vi "CreatePrivateEvents.vi"(8 "error in (no error)":errorcluster, 11 "ParseVectorFile":refnum<class "ParseVectorFile.lvclass">) -> (0 "error out":errorcluster, 3 "ParseVectorFile out":refnum<class "ParseVectorFile.lvclass">)   [LabVIEW 2019, in "ParseVectorFile.lvclass"]
doc: "---------------------------------------------------------------\nJKI State Machine Objects™\nhttp://jki.net/state-machine-objects/\nCopyright (C) 2005-2015, JKI <info@jki.net>\nALL RIGHTS RESERVEDJKI State Machine Objects (SMO) 1.0.0.4\nJKI - JKI\nCopyright (c) 2015, JKI"
uses:
  ParseVectorFile.lvclass
  Typedefs/PrivateEvents--ParseVectorFile.NewFile.ctl
  Typedefs/PrivateEvents--ParseVectorFile.New File Synchronous.ctl
  Typedefs/PublicEvents--ParseVectorFile.ParsedData.ctl
  ParsePaths/Path.lvclass
  Rectangle/Rectangle.lvclass
  Image/SVGImage.lvclass
  Dot/Dot.lvclass
  ParseVectorFile.lvclass/ParseVectorFile.ctl
  <vilib>/JKI/JKI SMO/SMO/SMO.lvclass
panel:
  # "For instructions on how to use the JKI State Machine Objects, examples and video tutorials, visit:\nhttp://jki.net/state-machine-objects/\n\nJKI State Machine Objects™\nhttp://jki.net/state-machine-objects/\nCopyright (C) 2005-2015, JKI <info@jki.net>\nALL RIGHTS RESERVED"
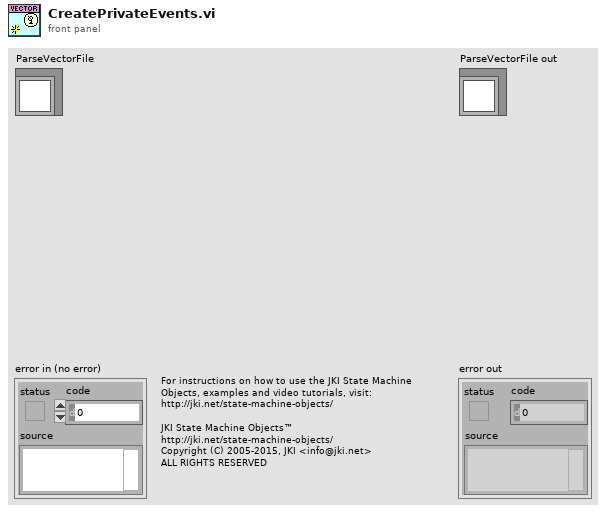
[diagram p1: front panel]
types:
  T1 = typedef "ParseVectorFile.lvclass/PrivateEvents--ParseVectorFile.New File Synchronous.ctl" = cluster{"Path":path, "Parsed Data":refnum<notifier>}
  T2 = typedef "ParseVectorFile.lvclass/PrivateEvents--ParseVectorFile.NewFile.ctl" = path
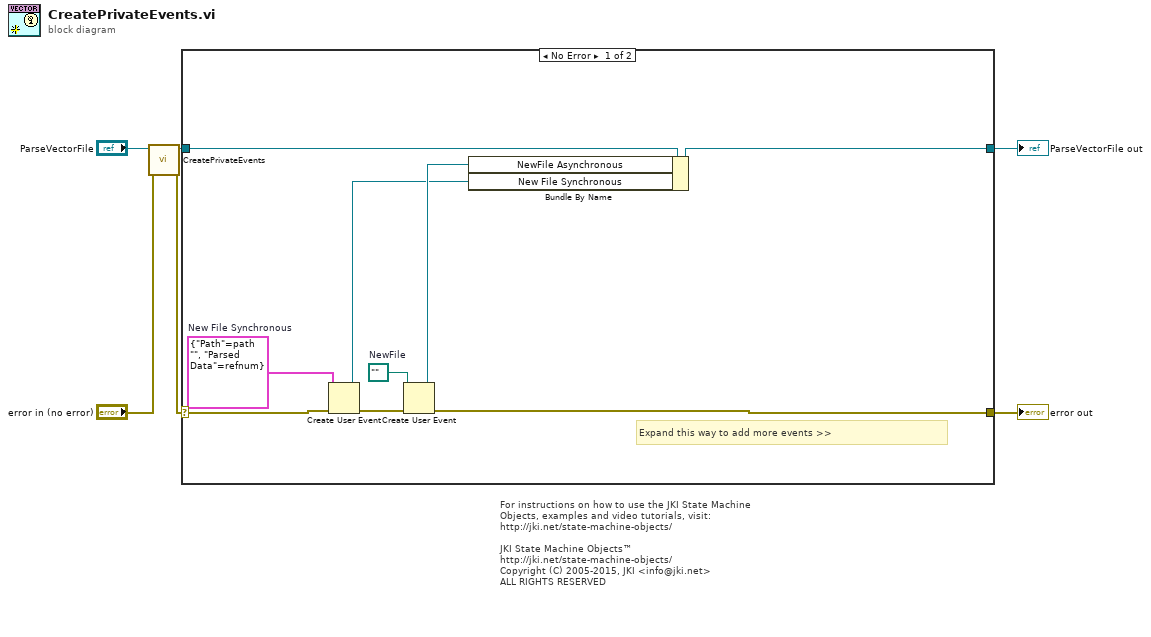
[diagram p0: block diagram]
diagram:
  # "For instructions on how to use the JKI State Machine Objects, examples and video tutorials, visit:\nhttp://jki.net/state-machine-objects/\n\nJKI State Machine Objects™\nhttp://jki.net/state-machine-objects/\nCopyright (C) 2005-2015, JKI <info@jki.net>\nALL RIGHTS RESERVED"
  n1 = call-parent "CreatePrivateEvents.vi"("error in (no error)"="error in (no error)", "SMO"="ParseVectorFile") -> ("error out"=w1:errorcluster, "SMO out"=w3:refnum<class "ParseVectorFile.lvclass">)  [unwired: 8 in]
  n2 = case shown="No Error" w1 {
    selector: w1 -> [w14 w17]
    tunnel: [w12 w17] -> w5
    tunnel: [w13 w16] -> w6
    tunnel: w3 -> [w15 w16]
    frame No Error {
      w8 = T1 {"Path"=path "", "Parsed Data"=refnum}  # New File Synchronous
      w11 = T2 path ""  # NewFile
      # "Expand this way to add more events >>"
      n3 = Create User Event(user event datatype=w8, error in=w14) -> (user event=w7:refnum<user-event>, error out=w9:errorcluster)
      n4 = Create User Event(user event datatype=w11, error in=w9) -> (user event=w10:refnum<user-event>, error out=w12:errorcluster)
      n5 = Bundle By Name(cluster=w15, "NewFile Asynchronous"=w10, "New File Synchronous"=w7) -> (w13:refnum<class "ParseVectorFile.lvclass">)
    }
    frame Error {
    }
  }
  "error out" <- w5
  "ParseVectorFile out" <- w6
